vi "Teardown.vi"(8 "error in (no error)":errorcluster, 11 "LUnit XML Report Test In":refnum<class "Text Report Test.lvclass">) -> (0 "error out":errorcluster, 3 "LUnit XML Report Test Out":refnum<class "Text Report Test.lvclass">)   [LabVIEW 2020, in "Text Report Test.lvclass"]
uses:
  Text Report Test.lvclass
  Text Report Test.lvclass/Text Report Test.ctl
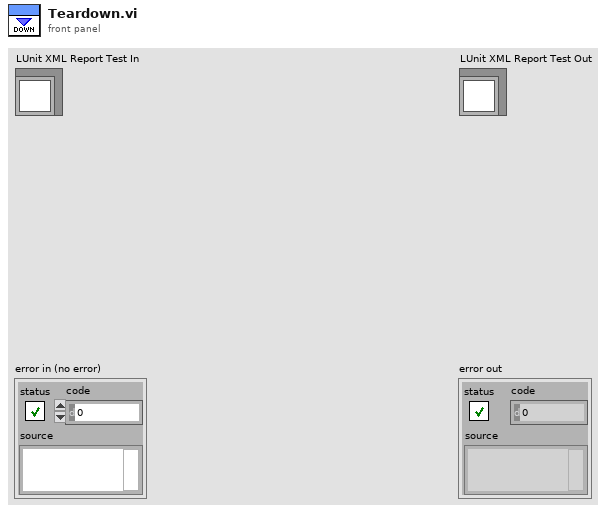
[diagram p1: front panel]
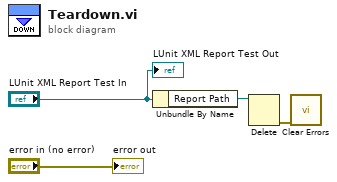
[diagram p0: block diagram]
diagram:
  n1 = Unbundle By Name("LUnit XML Report Test In") -> ("Report Path"=w1:path)
  n2 = Delete(path (use dialog)=w1) -> (error out=w2:errorcluster)  [unwired: 4 in, 2 out]
  n3 = call <vilib>:"Clear Errors.vi"("error in (no error)"=w2) -> ()  [unwired: 5 in, 2 out]
  "error out" <- "error in (no error)"
  "LUnit XML Report Test Out" <- "LUnit XML Report Test In"
